vi "CoordSystem_New.vi"(9 "PositiveZ":T1={"Axis"=[0.0, 0.0, 0.0]}, 10 "PositveY":T1={"Axis"=[0.0, 0.0, 0.0]}, 11 "PositiveX":T1={"Axis"=[0.0, 0.0, 0.0]}) -> (0 "Error":bool, 3 "out Coordinate System":T2={"Rotation"={"Q_quaternion"={"R"=1.0, "V"=[0.0, 0.0, 0.0]}}})   [LabVIEW 2019, in "Trajectory_Library.lvlib"]
doc: "Construct a Coordinte System data cluster which converts Pose3d objects between different standard coordinate frames. Contains a coordinate system with the given cardinal directions for each axis.\n\nInputs::\n -- PositiveX -- The cardinal direction of the positive x-axis.\n -- PositiveY -- The cardinal direction of the positive y-axis.\n -- PositiveZ -- The cardinal direction of the positive z-axis.\n\nReturns:\n -- out Coordinate System -- Data cluster containing the Coordinate System\n -- Error -- TRUE indicates an error occured."
uses:
  Trajectory_Library.lvlib
  TypeDef/COORDINATE_SYSTEM.ctl
  TypeDef/ROTATION3D.ctl
  TypeDef/QUATERNION.ctl
  TypeDef/COORDINATE_AXIS.ctl
  MatrixHelper_CoerceSize.vi
  Quaternion_Normalize.vi
  Quaternion_New_Default.vi
  <vilib>/Analysis/7linalg.llb/Create Special Matrix.vi
  <vilib>/Analysis/7linalg.llb/Create Special Real Matrix.vi
  <vilib>/Analysis/Matrix/Numeric/Conversions/Array To Matrix - RA.vi
  <vilib>/Analysis/Matrix/NI_Matrix.lvlib
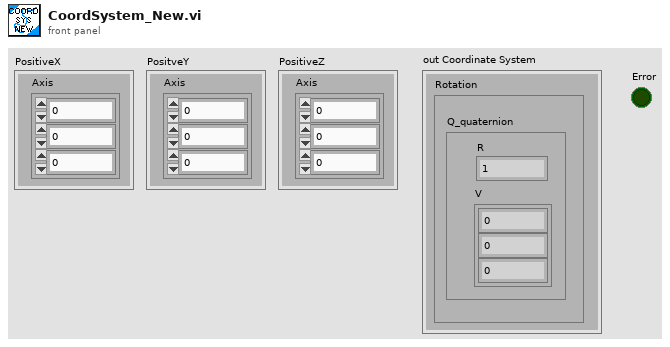
[diagram p1: front panel]
types:
  T1 = typedef "Trajectory_Library.lvlib/COORDINATE_AXIS.ctl" = cluster{"Axis":dbl[]}
  T2 = typedef "Trajectory_Library.lvlib/COORDINATE_SYSTEM.ctl" = cluster{"Rotation":T3}
  T3 = typedef "Trajectory_Library.lvlib/ROTATION3D.ctl" = cluster{"Q_quaternion":T4}
  T4 = typedef "Trajectory_Library.lvlib/QUATERNION.ctl" = cluster{"R":dbl, "V":dbl[]}
  T5 = typedef "NI_Matrix.lvlib/RealMatrix.ctl" = dbl[][]
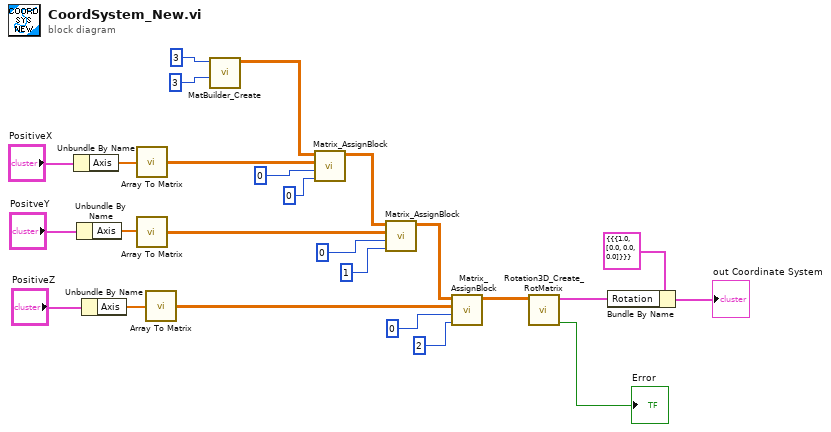
[diagram p0: block diagram]
diagram:
  n1 = Unbundle By Name("PositiveX") -> ("Axis"=w15:dbl[])
  n2 = Unbundle By Name("PositveY") -> ("Axis"=w14:dbl[])
  n3 = Unbundle By Name("PositiveZ") -> ("Axis"=w13:dbl[])
  n4 = call-poly <vilib>:"Array To Matrix.vi"("Real 1D Array"=w15) -> ("Real Matrix (Column Vector)"=w12:T5)
  n5 = call-poly <vilib>:"Array To Matrix.vi"("Real 1D Array"=w14) -> ("Real Matrix (Column Vector)"=w11:T5)
  n6 = call-poly <vilib>:"Array To Matrix.vi"("Real 1D Array"=w13) -> ("Real Matrix (Column Vector)"=w10:T5)
  n7 = call "MatBuilder_Create.vi"("Columns"=3, "Rows"=3) -> ("output matrix"=w21:T5)  [unwired: 9 in]
  n8 = call "Matrix_AssignBlock.vi"("StartColumn"=0, "StartRow"=0, "Other Matrix"=w12, "input matrix"=w21) -> ("output matrix"=w20:T5)  [unwired: 7 in]
  n9 = call "Matrix_AssignBlock.vi"("StartColumn"=1, "StartRow"=0, "Other Matrix"=w11, "input matrix"=w20) -> ("output matrix"=w19:T5)  [unwired: 7 in]
  n10 = call "Matrix_AssignBlock.vi"("StartColumn"=2, "StartRow"=0, "Other Matrix"=w10, "input matrix"=w19) -> ("output matrix"=w3:T5)  [unwired: 7 in]
  n11 = call "Rotation3D_Create_RotMatrix.vi"("RotationMatrix"=w3) -> ("Error"=→"Error":bool, "Rotation3d"=w1:T3)  [unwired: 9 in]
  n12 = Bundle By Name(cluster=T2 {"Rotation"={"Q_quaternion"={"R"=1.0, "V"=[0.0, 0.0, 0.0]}}} ("sumPOSE"), "Rotation"=w1) -> (→"out Coordinate System":T2)
